vi "Query UL-DL Pattern.vi"(8 "error in (no error)":errorcluster, 9 "SCS (30 kHz)":i32(ring)=1 items=["15 kHz", "30 kHz", "60 kHz"], 10 "Instance (1)":T1=1, 11 "VISA resource name":refnum<visa-resource-name>) -> (0 "error out":errorcluster, 1 "No Of DL Symbols":i32, 2 "No Of DL Slots":i32, 3 "VISA resource name out":refnum<visa-resource-name>, 4 "No Of UL Slots":i32, 5 "No Of UL Symbols":i32)   [LabVIEW 2020, in "Rohde&Schwarz CMWXP NR FR1 Measurement.lvlib"]
doc: "Retrives the UL-DL pattern for the <SCSpacing>.\n\nAttribute:\n-\n\nRemote-control command:\nCONFigure:NRSub:MEAS<i>:ULDL:PATTern?"
uses:
  <instrlib>/Rohde&Schwarz CMWXP NR FR1 Measurement/Rohde&Schwarz CMWXP NR FR1 Measurement.lvlib
  <instrlib>/Rohde&Schwarz CMWXP NR FR1 Measurement/Private/_Instance.ctl
  <instrlib>/Rohde&Schwarz CMWXP NR FR1 Measurement/Private/rsidr_core.llb/rsidr_core.lvlib
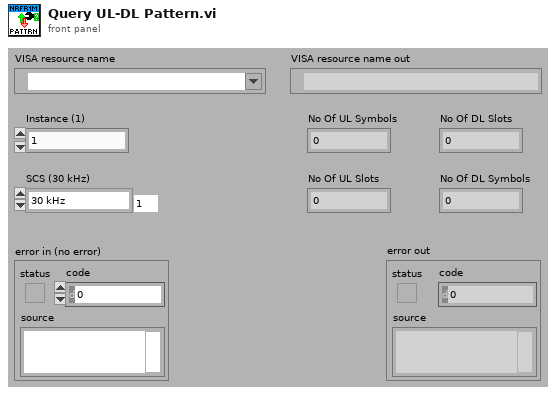
[diagram p1: front panel]
types:
  T1 = typedef "Rohde&Schwarz CMWXP NR FR1 Measurement.lvlib/_Instance.ctl" = i32
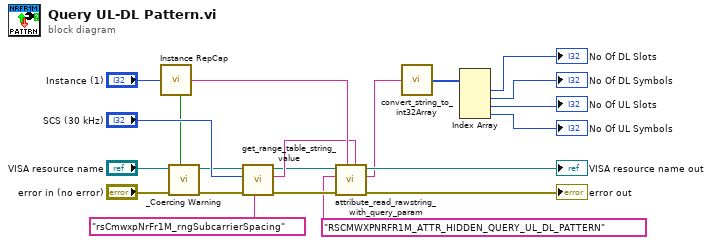
[diagram p0: block diagram]
diagram:
  n1 = call <instrlib>:"Instance RepCap.vi"("Instance In"="Instance (1)") -> ("In Range?"=w1:bool, "RepCap Identifier Out"=w14:string)  [unwired: 1 in]
  n2 = call <instrlib>:"_Coercing Warning.vi"("In Range?"=w1, "error in (no error)"="error in (no error)", "VISA resource name"="VISA resource name") -> ("error out"=w3:errorcluster, "VISA resource name out"=w2:refnum<visa-resource-name>)  [unwired: 7 in]
  n3 = call <instrlib>:"get_range_table_string_value.vi"("Range Table ID in"="rsCmwxpNrFr1M_rngSubcarrierSpacing", "error in"=w3, "I32 input"="SCS (30 kHz)", "VISA resource name"=w2) -> ("error out"=w12:errorcluster, "String Value out"=w13:string, "VISA resource name out"=w11:refnum<visa-resource-name>)  [unwired: 5 in]
  n4 = call <instrlib>:"attribute_read_rawstring_with_query_param.vi"("Query Parameter (None)"=w13, "Repeated Capability"=w14, "error in"=w12, "Attribute ID"="RSCMWXPNRFR1M_ATTR_HIDDEN_QUERY_UL_DL_PATTERN", "VISA resource name"=w11) -> ("error out"=→"error out":errorcluster, "Raw String out"=w7:string, "VISA resource name out"=→"VISA resource name out":refnum<visa-resource-name>)  [unwired: 4 in]
  n5 = call <instrlib>:"convert_string_to_int32Array.vi"("string in"=w7) -> ("int32 array out"=w19:i32[])  [unwired: 3 in, 1 out]
  n6 = Index Array(array=w19) -> (element #1=→"No Of DL Slots":i32, element #2=→"No Of DL Symbols":i32, element #3=→"No Of UL Slots":i32, element #4=→"No Of UL Symbols":i32)  [unwired: 4 in]
